vi "Line Detector Peak Finder.vi"(6 "Spectrum Recorder Configuration":T1={"Start frequency"=500000.0, "End frequency"=2000000.0, "Coarse step"=100.0, "Step duration"=0.004, "Red Pitaya address"="192.168.1.100", "Open plot \non start"=FALSE, "Regions width"=2000.0, "Fine step"=1.0, "Pause between scans"=0.0, "Clear rgs on start"=FALSE, "Output amplitude"=1.0} {"Output amplitude" min=0.0 max=1.0 step=0.1 format="%#_6pV"; "Pause between scans" format="%#_6ps"; "Fine step" min=0.001 format="%#_6pHz"; "Regions width" format="%#_6pHz"; "Step duration" format="%#_6ps"; "Coarse step" format="%#_6pHz"; "End frequency" format="%#_6pHz"; "Start frequency" format="%#_6pHz"}, 7 "Frequency":dbl[](array[numeric]), 8 "error in (no error)":errorcluster, 9 "Valid Spectrum Recorder Configuration":bool, 10 "Signal":cdb[](array[numeric]), 11 "Line Detector Configuration":T2={"Peak width guess"=500.0, "Background removal"=enum."High-pass", "Smoothing"=enum."Low-pass", "Smooth window"=200.0, "Relative threshold"=0.2, "Finder algorithm"=enum."Wavelet", "Bgd window"=50000.0, "Spectrum recorder module name"="Spectrum Recorder", "Fit window"=1000.0, "Initial fit guess"=enum."Peak finder", "Follow\npeaks"=FALSE, "Re-sample"=nan} {"Re-sample" format="%#_6pHz"; "Fit window" format="%#_6pHz"; "Bgd window" format="%#_6pHz"; "Smooth window" format="%#_6pHz"; "Peak width guess" format="%#_6pHz"}) -> (0 "error out":errorcluster, 1 "Peak Plot":cluster{"Ramp Pattern":dbl[], "X":dbl[]}[](graph), 2 "Initial fit guess":dbl[][](array[numeric]) format="%#_4p", 3 "Regions frequencies":waveform(dbl)[](array[waveform]), 4 "Regions signals":waveform(cdb)[](array[waveform]), 5 "Peaks":dbl[](array[numeric]) format="%#_4p")   [LabVIEW 2016]
uses:
  LabActor/Post-Processors/Line Detector/Resonance Detector Configuration.ctl
  Red Pitaya/RP Core/Red Pitaya Transceiver Driver/Spectrum Configuration.ctl
panel:
  # "F0         dF     Ampl   Phase   Xbgrd   Ybgrd"
  # "Peak finder config"
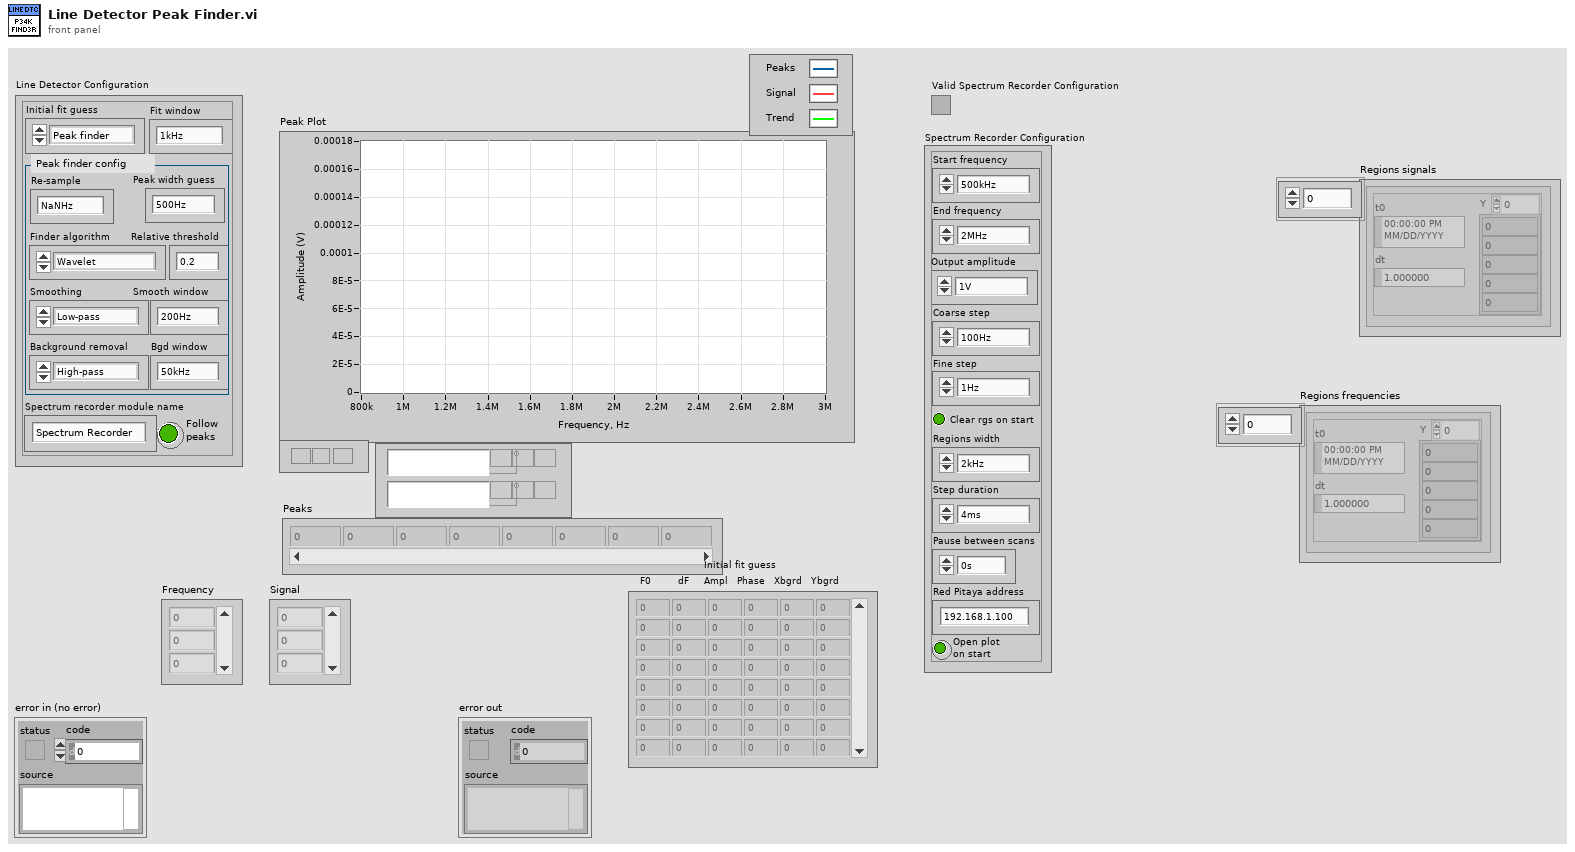
[diagram p1: front panel]
types:
  T1 = typedef "Spectrum Configuration.ctl" = cluster{"Start frequency":dbl, "End frequency":dbl, "Coarse step":dbl, "Step duration":dbl, "Red Pitaya address":string, "Open plot \non start":bool, "Regions width":dbl, "Fine step":dbl, "Pause between scans":dbl, "Clear rgs on start":bool, "Output amplitude":dbl}
  T2 = typedef "Resonance Detector Configuration.ctl" = cluster{"Peak width guess":dbl, "Background removal":enum16{"NONE", "High-pass", "Detrend"}, "Smoothing":enum16{"NONE", "Low-pass", "Denoise"}, "Smooth window":dbl, "Relative threshold":dbl, "Finder algorithm":enum16{"Basic", "Wavelet", "Wavelet+detrend"}, "Bgd window":dbl, "Spectrum recorder module name":string, "Fit window":dbl, "Initial fit guess":enum16{"Peak finder", "Last fit"}, "Follow\npeaks":bool, "Re-sample":dbl}
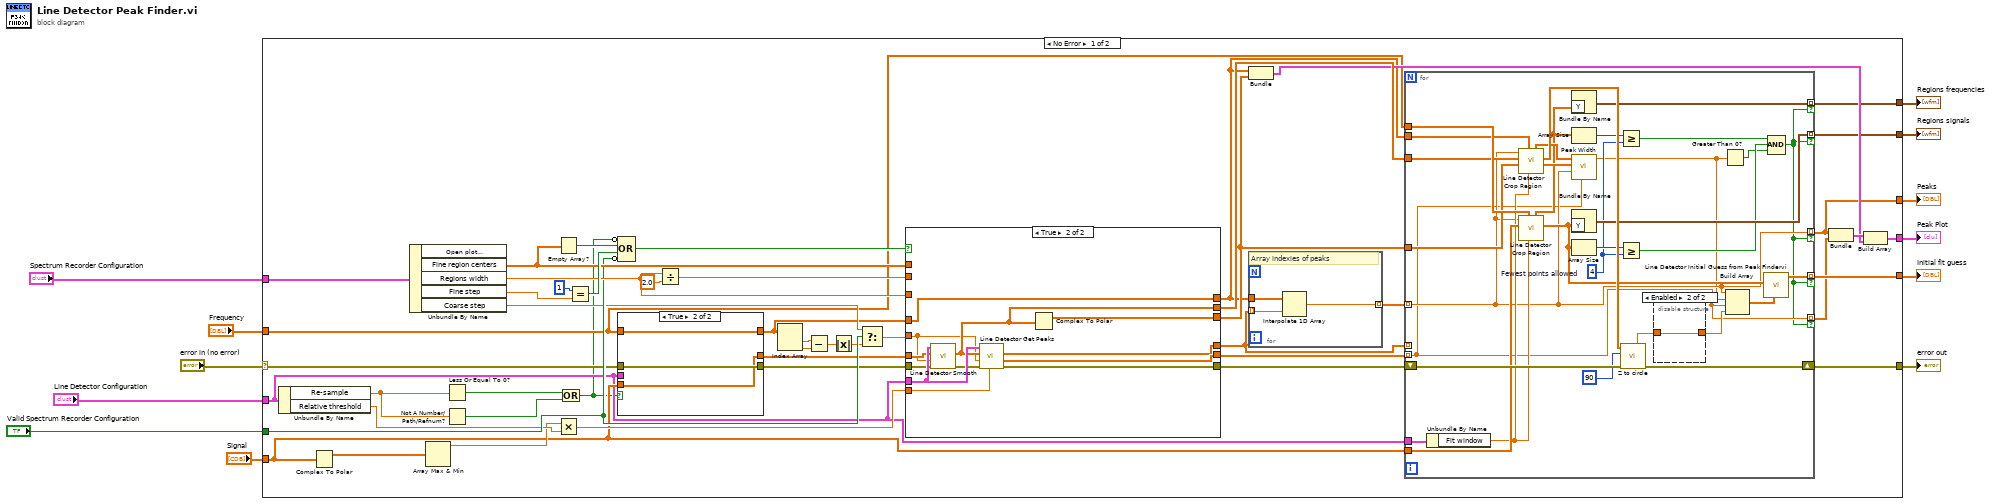
[diagram p0: block diagram]
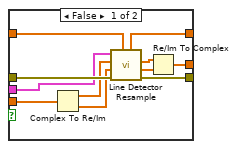
[diagram p2: hidden frame]
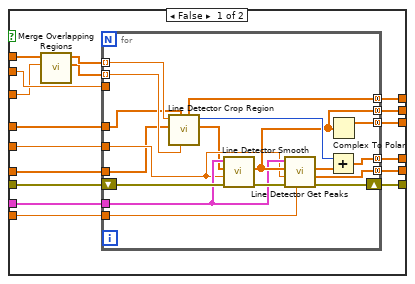
[diagram p3: hidden frame]
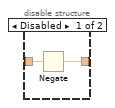
[diagram p4: hidden frame]
diagram:
  n1 = case shown="No Error" "error in (no error)" {
    selector: "error in (no error)" -> [w25 w159]
    tunnel: "Line Detector Configuration" -> [w21 _]
    tunnel: [w58 w159] -> w10
    tunnel: [w60 _] -> w9
    tunnel: [w14 _] -> w8
    tunnel: "Frequency" -> [w20 _]
    tunnel: "Signal" -> [w23 _]
    tunnel: "Spectrum Recorder Configuration" -> [w54 _]
    tunnel: "Valid Spectrum Recorder Configuration" -> [w39 _]
    tunnel: [w41 _] -> w3
    tunnel: [w16 _] -> w2
    tunnel: [w15 _] -> w1
    frame No Error {
      n2 = Unbundle By Name(w21) -> ("Re-sample"=w28:dbl, "Relative threshold"=w32:dbl)
      n3 = Complex To Polar(r * e^(i*theta)=w23) -> (r=w30:dbl[])  [unwired: 1 out]
      n4 = Unbundle By Name(w54) -> ("Fine region centers"=w47:dbl[], "Regions width"=w43:dbl, "Fine step"=w51:dbl, "Coarse step"=w38:dbl)  [unwired: 1 out]
      n5 = Array Max & Min(array=w30) -> (max value=w31:dbl)  [unwired: 3 out]
      n6 = Less Or Equal To 0?(x=w28) -> (x <= 0?=w27:bool)
      n7 = Not A Number/Path/Refnum?(number/path/refnum=w28) -> (NaN/Path/Refnum?=w26:bool)
      n8 = Empty Array?(array=w47) -> (empty?=w50:bool)
      n9 = Multiply(x=w31, y=w32) -> (x*y=w29:dbl)
      n10 = Or(x=w27, y=w26) -> (x .or. y?=w19:bool)
      n11 = Equal?(x=1, y=w51) -> (x = y?=w53:bool)
      n12 = Compound Arithmetic op=OR(invert w19, w50, w53, invert w39) -> (w49:bool)
      n13 = case shown="True" w19 {
        tunnel: w25 -> [w71 w74]
        tunnel: [w70 w74] -> w24
        tunnel: w23 -> [w69 w73]
        tunnel: [w64 w73] -> w22
        tunnel: w21 -> [w63 _]
        tunnel: w20 -> [w62 w72]
        tunnel: [w61 w72] -> w18
        frame False {
          n14 = Complex To Re/Im(x + iy=w69) -> (x=w68:dbl[], y=w67:dbl[])
          n15 = call "Line Detector Resample.vi"("Frequency"=w62, "error in (no error)"=w71, "Signal Y"=w67, "Signal X"=w68, "Line Detector Configuration"=w63) -> ("error out"=w70:errorcluster, "Signal Y out"=w65:dbl[], "Signal X out"=w66:dbl[], "Frequency out"=w61:dbl[])  [unwired: 3 in]
          n16 = Re/Im To Complex(1:w65, 2:w66) -> (0:w64:cdb[])
        }
        frame True {
        }
      }
      n17 = Divide(x=w43, y=2.0) -> (x/y=w45:dbl)
      n18 = Index Array(array=w18) -> (element #1=w37:dbl, element #2=w36:dbl)  [unwired: 2 in]
      n19 = Subtract(x=w37, y=w36) -> (x-y=w35:dbl)
      n20 = Absolute Value(x=w35) -> (abs(x)=w34:dbl)
      n21 = Select(t=w38, s=w39, f=w34) -> (s? t:f=w33:dbl)
      n22 = case shown="True" w49 {
        tunnel: [w87 w118] -> w40
        tunnel: [w94 w124] -> w59
        tunnel: w21 -> [w93 w123]
        tunnel: [w92 w122] -> w57
        tunnel: [w91 w121] -> w55
        tunnel: w24 -> [w90 w120]
        tunnel: w18 -> [w89 w114]
        tunnel: w22 -> [w88 w119]
        tunnel: w47 -> [w81 _]
        tunnel: w45 -> [w86 _]
        tunnel: w33 -> [w85 w117]
        tunnel: [w84 w114] -> w17
        tunnel: [w83 w116] -> w42
        tunnel: w43 -> [w82 _]
        tunnel: w29 -> [w78 w113]
        frame False {
          n23 = call "Merge Overlapping Regions.vi"("Regions width"=w82, "Region centers"=w81) -> ("Region widths out"=w79:dbl[], "Region centers out"=w80:dbl[])  [unwired: 8 in]
          n24 = for {
            tunnel: [w98] -> w94 mode=concatenating
            tunnel: w93 -> [w102]
            tunnel: [w103] -> w91 mode=concatenating
            tunnel: w89 -> [w109]
            tunnel: w88 -> [w96]
            tunnel: [w107] -> w87 mode=concatenating
            shift-right: [w100] -> w92
            shift-left: w90 -> [w105]
            tunnel: w80 -> [w111] mode=indexing
            tunnel: w86 -> [_]
            tunnel: w85 -> [w101]
            tunnel: [w108] -> w84 mode=concatenating
            tunnel: [w112] -> w83 mode=concatenating
            tunnel: w79 -> [w110] mode=indexing
            tunnel: w78 -> [w97]
            n25 = call "Line Detector Crop Region.vi"("Region width"=w110, "Frequency"=w109, "Signal"=w96, "Center frequency"=w111) -> ("Signal  out"=w95:cdb[], "Start index"=w106:i32, "Frequency out"=w108:dbl[])  [unwired: 4 in, 1 out]
            n26 = call "Line Detector Smooth.vi"("error in (no error)"=w105, "Frequency step"=w101, "Signal"=w95, "Line Detector Configuration"=w102) -> ("error out"=w104:errorcluster, "Signal out"=w103:cdb[])  [unwired: 6 in]
            n27 = call "Line Detector Get Peaks.vi"("Threshold"=w97, "error in (no error)"=w104, "Frequency step"=w101, "Signal"=w103, "Line Detector Configuration"=w102) -> ("error out"=w100:errorcluster, "Peak amplitudes"=w98:dbl[], "Peak locations"=w99:dbl[])  [unwired: 4 in]
            n28 = Add(x=w106, y=w99) -> (x+y=w107:dbl[])
            n29 = Complex To Polar(r * e^(i*theta)=w103) -> (r=w112:dbl[])  [unwired: 1 out]
          }
        }
        frame True {
          n30 = call "Line Detector Smooth.vi"("error in (no error)"=w120, "Frequency step"=w117, "Signal"=w119, "Line Detector Configuration"=w123) -> ("error out"=w115:errorcluster, "Signal out"=w121:cdb[])  [unwired: 6 in]
          n31 = call "Line Detector Get Peaks.vi"("Threshold"=w113, "error in (no error)"=w115, "Frequency step"=w117, "Signal"=w121, "Line Detector Configuration"=w123) -> ("error out"=w122:errorcluster, "Peak amplitudes"=w124:dbl[], "Peak locations"=w118:dbl[])  [unwired: 4 in]
          n32 = Complex To Polar(r * e^(i*theta)=w121) -> (r=w116:dbl[])  [unwired: 1 out]
        }
      }
      n33 = Bundle("Frequency"=w17, w42) -> (w44:cluster{"Frequency":dbl[], dbl[]})  [unwired: 1 in]
      n34 = for {
        tunnel: w17 -> [w77]
        tunnel: w40 -> [w76] mode=indexing
        tunnel: [w75] -> w48 mode=indexing
        # "Array indexies of peaks"
        n35 = Interpolate 1D Array(1:w76, 2:w77) -> (0:w75:dbl)
      }
      n36 = for {
        tunnel: w20 -> [w148]
        tunnel: w23 -> [w147]
        tunnel: w40 -> [_] mode=indexing
        tunnel: w59 -> [w128] mode=indexing
        tunnel: w21 -> [w149]
        shift-right: [w150] -> w58
        shift-left: w57 -> [w155]
        tunnel: w48 -> [w129] mode=indexing
        tunnel: w42 -> [w142]
        tunnel: w55 -> [w143]
        tunnel: [w139] -> w41 mode=indexing if=w127
        tunnel: w17 -> [w145]
        tunnel: [w138] -> w16 mode=indexing if=w127
        tunnel: [w137] -> w15 mode=indexing if=w127
        tunnel: [w129] -> w14 mode=indexing if=w127
        tunnel: [w128] -> w13 mode=indexing if=w127
        w132 = 4  # Fewest points allowed
        n37 = Unbundle By Name(w149) -> ("Fit window"=w146:dbl)
        n38 = call "Line Detector Crop Region.vi"("Region width"=w146, "Frequency"=w145, "Magnitude"=w142, "Signal"=w143, "Center frequency"=w129) -> ("Magnitude out"=w141:dbl[], "Signal  out"=w144:cdb[], "Frequency out"=w140:dbl[])  [unwired: 3 in, 1 out]
        n39 = call "Line Detector Crop Region.vi"("Region width"=w146, "Frequency"=w148, "Signal"=w147, "Center frequency"=w129) -> ("Signal  out"=w136:cdb[], "Frequency out"=w135:dbl[])  [unwired: 4 in, 2 out]
        n40 = Bundle By Name("Y"=w135) -> (w137:waveform(dbl))  [unwired: 1 in]
        n41 = Array Size(array=w135) -> (size(s)=w134:i32)
        n42 = call "Peak Width.vi"("Peak Y"=w128, "Peak X"=w129, "Y"=w141, "X"=w140) -> ("width"=w126:dbl)  [unwired: 5 in, 2 out]
        n43 = Bundle By Name("Y"=w136) -> (w138:waveform(cdb))  [unwired: 1 in]
        n44 = Array Size(array=w136) -> (size(s)=w133:i32)
        n45 = Greater Or Equal?(x=w134, y=w132) -> (x >= y?=w131:bool)
        n46 = Greater Or Equal?(x=w133, y=w132) -> (x >= y?=w130:bool)
        n47 = call "Z to circle.vi"("Error In"=w155, "Plot points"=90, "Z"=w144) -> ("Error Out"=w150:errorcluster, "theta"=w153:dbl)  [unwired: 2 in, 5 out]
        n48 = disable-structure shown="Enabled" {
          disable-tunnel: w153 -> [w157 w158]
          disable-tunnel: [w156 w158] -> w152
          frame Disabled {
            n49 = Negate(x=w157) -> (-x=w156:dbl)
          }
          frame Enabled {
          }
        }
        n50 = Greater Than 0?(x=w126) -> (x > 0?=w125:bool)
        n51 = Build Array(w129, w126, w128, w152) -> (w151:dbl[])
        n52 = call "Line Detector Initial Guess from Peak Findervi.vi"("Peak finder guess"=w151, "Signal"=w136) -> ("Initial guess"=w139:dbl[])  [unwired: 9 in]
        n53 = Compound Arithmetic op=AND(w131, w130, w125) -> (w127:bool)
      }
      n54 = Bundle(w14, w13) -> (w56:cluster{dbl[], dbl[]})  [unwired: 1 in]
      n55 = Build Array(w56, w44) -> (w60:cluster{"Frequency":dbl[], dbl[]}[])
    }
    frame Error {
    }
  }
  "error out" <- w10
  "Peak Plot" <- w9
  "Peaks" <- w8
  "Initial fit guess" <- w3
  "Regions signals" <- w2
  "Regions frequencies" <- w1
